vi "Run Time Mode.vi"(8 "error in (no error)":errorcluster caption="entrée d'erreur (pas d'erreur)", 10 "Refnum VI":refnum<vi>, 11 "UI Cam Basler en entrée":refnum<class "UI Cam Basler.lvclass">) -> (0 "error out":errorcluster caption="sortie d'erreur", 3 "UI Cam Basler en sortie":refnum<class "UI Cam Basler.lvclass">)   [LabVIEW 2023, in "UI Cam Basler.lvclass"]
uses:
  UI Cam Basler.lvclass
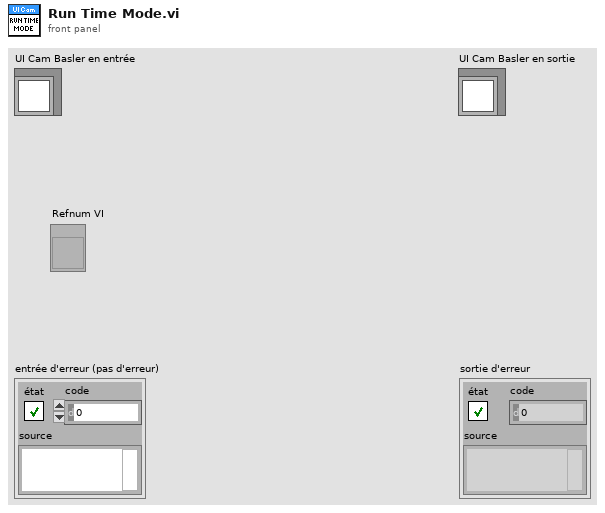
[diagram p1: front panel]
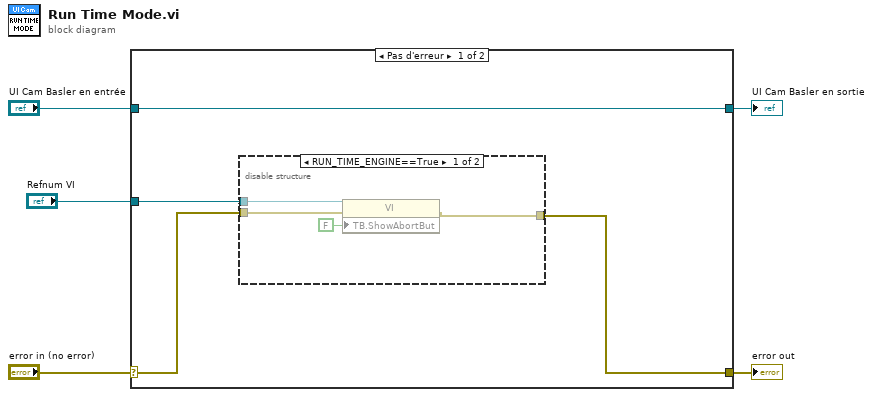
[diagram p0: block diagram]
diagram:
  n1 = case shown="Pas d'erreur" "error in (no error)" {
    selector: "error in (no error)" -> [w7 w15]
    tunnel: [w6 w15] -> w4
    tunnel: [w9 w14] -> w2
    tunnel: "UI Cam Basler en entrée" -> [w9 w14]
    tunnel: "Refnum VI" -> [w8 _]
    frame No Error {
      n2 = disable-structure shown="RUN_TIME_ENGINE==True" {
        disable-tunnel: w8 -> [w13 _]
        disable-tunnel: w7 -> [w11 _]
        disable-tunnel: [w10 _] -> w6
        frame condition #0 {
          n3 = property class="VI"(reference=w13, error in=w11, "TB.ShowAbortBut"=FALSE ("Barre d'outils:Bouton Abandonner")) -> (error out=w10:errorcluster)  [unwired: 1 out]
        }
        frame condition #1 (active) {
        }
      }
    }
    frame Error {
    }
  }
  "error out" <- w4
  "UI Cam Basler en sortie" <- w2
